vi "Insert VI.vi"(8 "error in (no error)":errorcluster, 10 "sub panel":refnum<vi>, 11 "Logger in":refnum<class "Logger.lvclass">) -> (0 "error out":errorcluster, 3 "Logger out":refnum<class "Logger.lvclass">)   [LabVIEW 2020, in "Logger.lvlib" / "Logger.lvclass"]
uses:
  Logger.lvclass
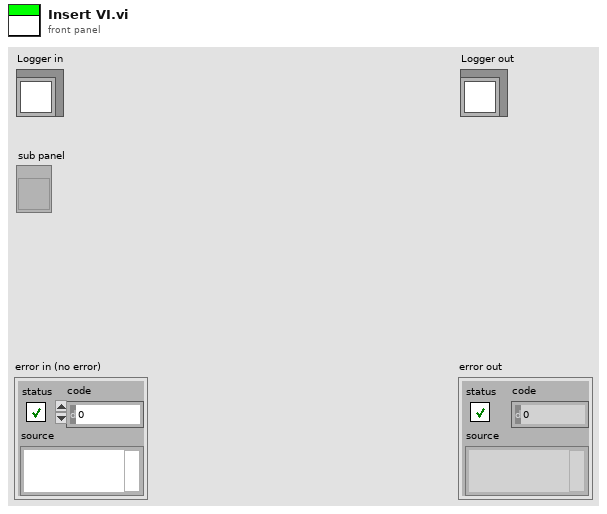
[diagram p1: front panel]
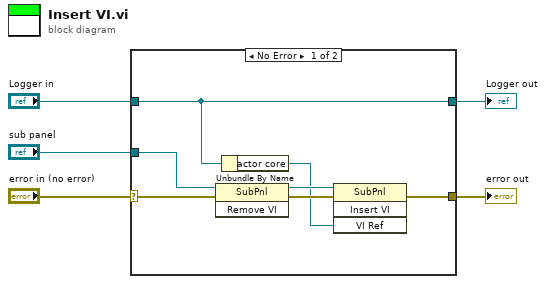
[diagram p0: block diagram]
diagram:
  n1 = case shown="No Error" "error in (no error)" {
    selector: "error in (no error)" -> [w12 w14]
    tunnel: [w6 w14] -> w4
    tunnel: [w8 w13] -> w2
    tunnel: "Logger in" -> [w8 w13]
    tunnel: "sub panel" -> [w11 _]
    frame No Error {
      n2 = invoke class="SubPnl" method="Remove VI"(reference=w11, error in=w12) -> (reference out=w9:refnum<vi>, error out=w10:errorcluster)  [unwired: 1 in, 1 out]
      n3 = Unbundle By Name(w8) -> ("actor core"=w7:refnum<vi>)
      n4 = invoke class="SubPnl" method="Insert VI"(reference=w9, error in=w10, "VI Ref"=w7) -> (error out=w6:errorcluster)  [unwired: 1 in, 3 out]
    }
    frame Error {
    }
  }
  "error out" <- w4
  "Logger out" <- w2
